vi "Angle_around_Y_axis.vi"(1 "gy":dbl, 2 "dt":dbl=0.1 format="%#_13g") -> (0 "Angle around the Y-axis (*roll)":dbl)   [LabVIEW 2015]
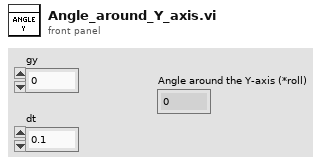
[diagram p1: front panel]
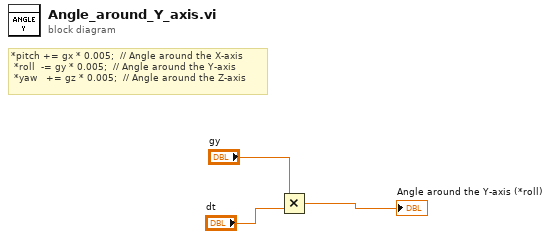
[diagram p0: block diagram]
diagram:
  # "*pitch += gx * 0.005;  // Angle around the X-axis\n *roll  -= gy * 0.005;  // Angle around the Y-axis\n *yaw   += gz * 0.005;  // Angle around the Z-axis"
  n1 = Multiply(x="gy", y="dt") -> (x*y=→"Angle around the Y-axis (*roll)":dbl)
